vi "Sequencers.vi"() -> ()   [LabVIEW 2019]
panel:
  in  "Elevator Limit Switch":bool
  in  "Adam Smashing the button":bool
  out "Piston 3":bool
  out "Timer Value":i32
  out "Sequencer Step":i32
  out "Piston 2":bool
  out "Piston 1":bool
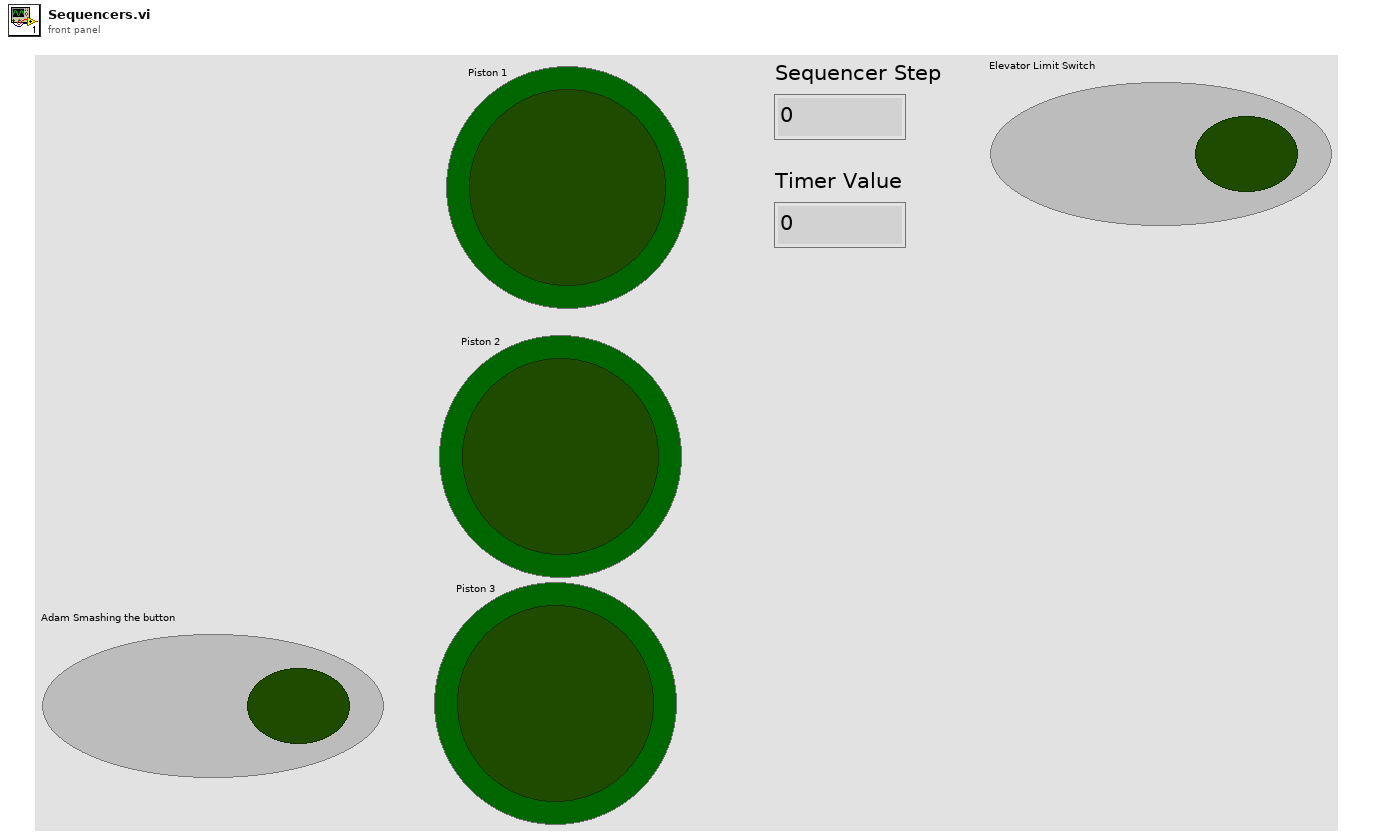
[diagram p1: front panel]
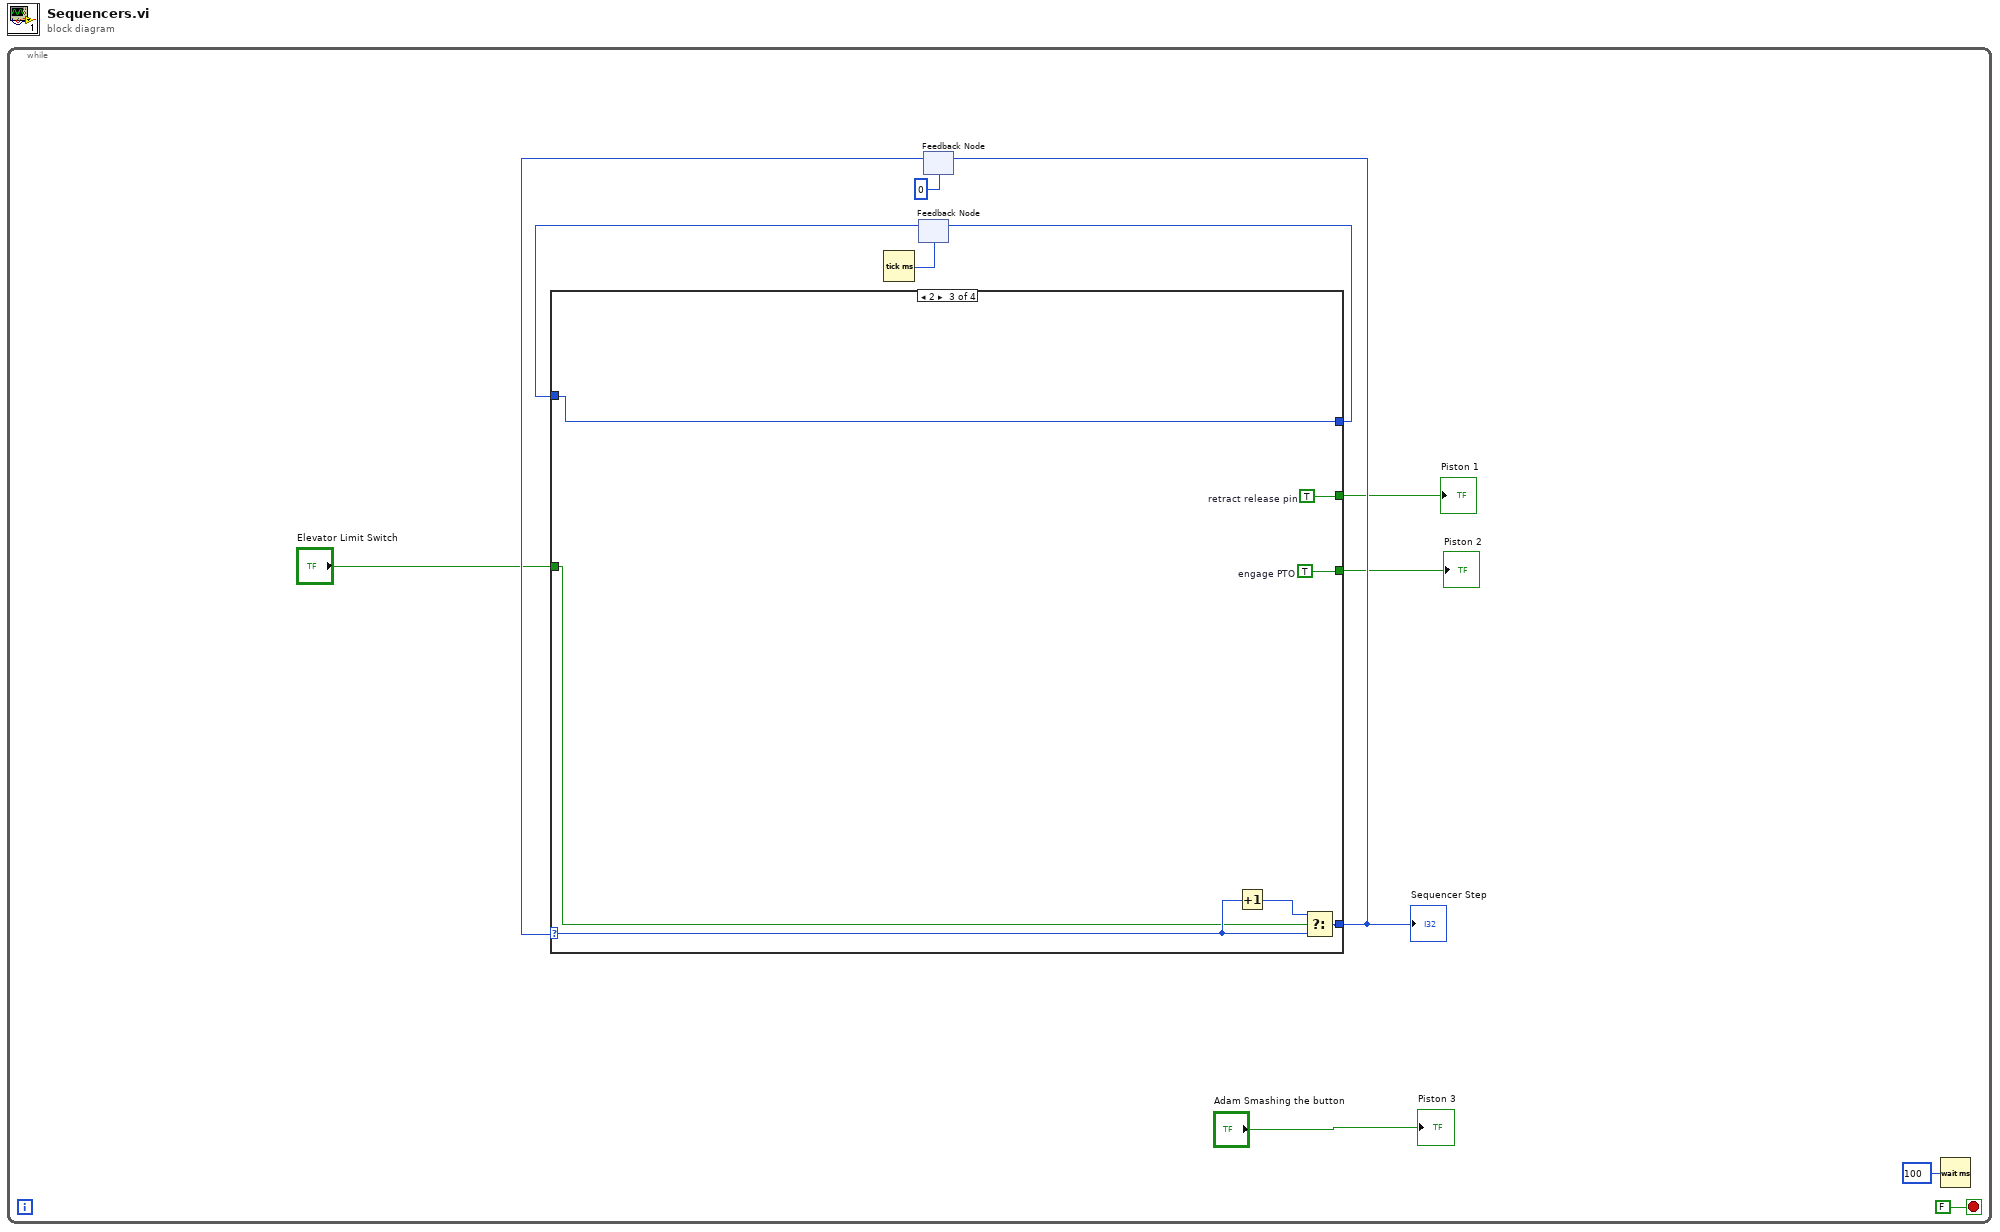
[diagram p0: block diagram]
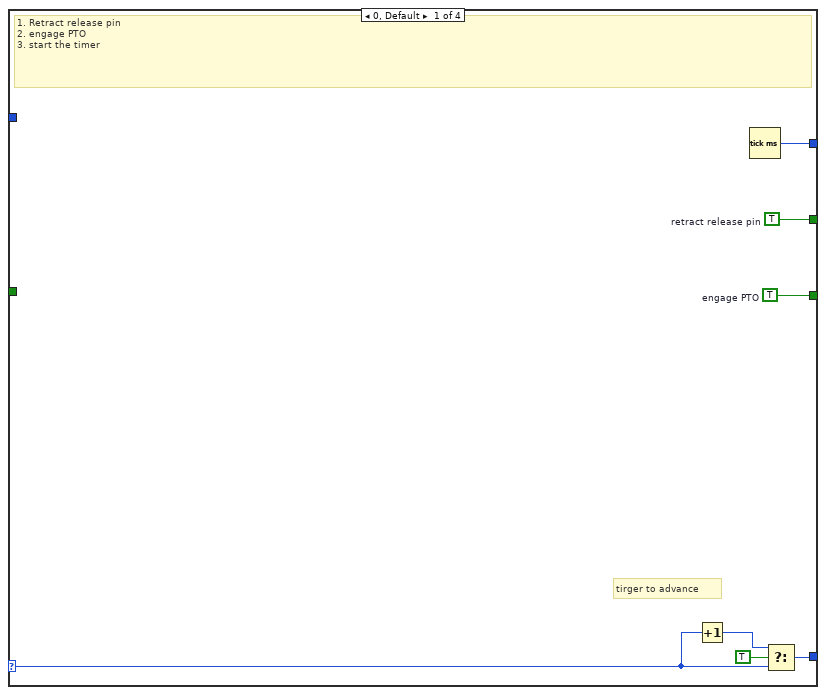
[diagram p2: hidden frame]
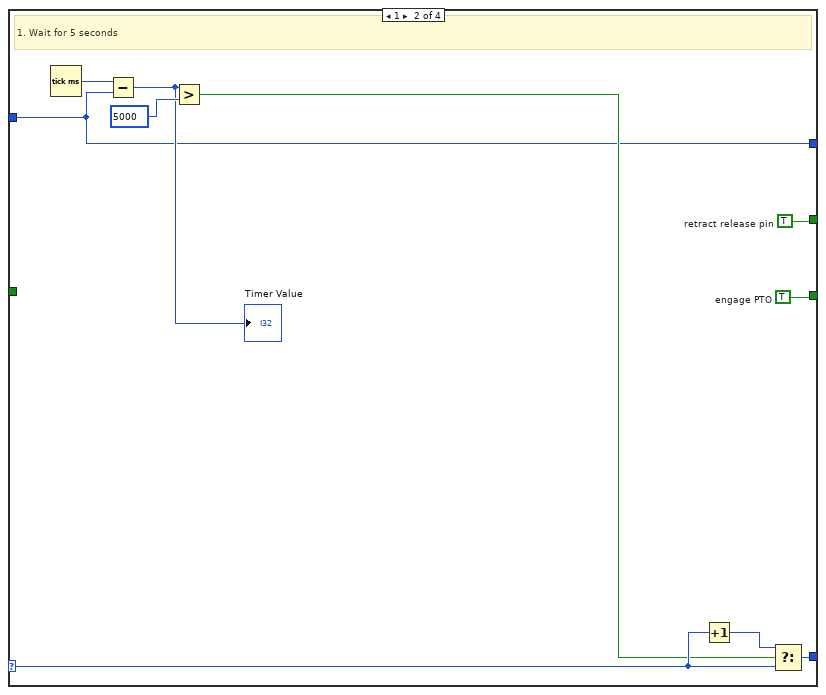
[diagram p3: hidden frame]
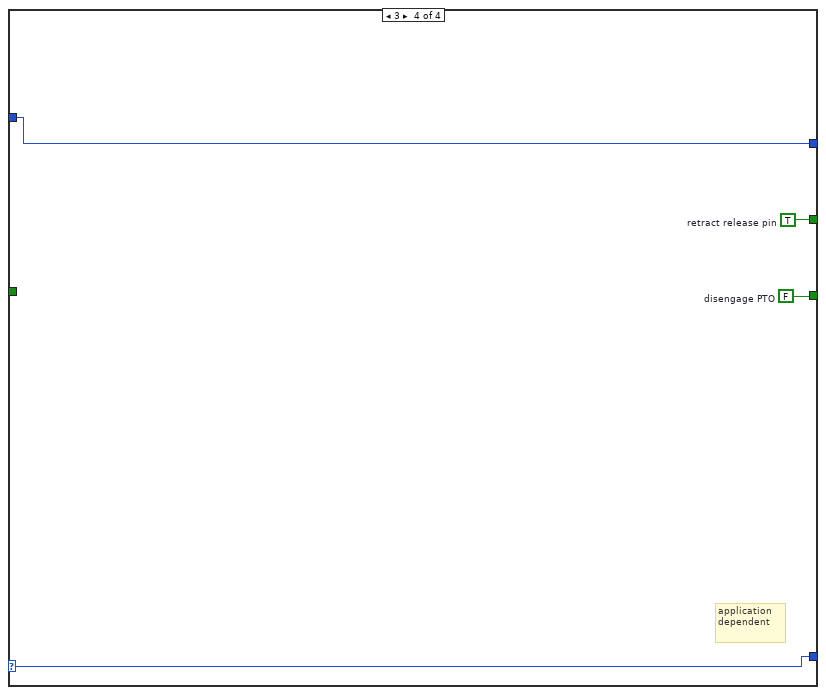
[diagram p4: hidden frame]
diagram:
  n1 = while {
    stop <- FALSE stop-if-true
    n2 = Tick Count (ms)() -> (millisecond timer value=w3:u32)
    n3 = feedback #1(w3) -> (w5:u32)
    n4 = feedback #2(0) -> (w11:i32)
    n5 = case shown="2" w11 {
      selector: w11 -> [w18 w28 w35 w40]
      tunnel: [w19 w27 w34 w40] -> w10
      tunnel: [w16 w26 w33 w39] -> w7
      tunnel: [w15 w25 w32 w38] -> w6
      tunnel: [w13 w20 w31 w37] -> w4
      tunnel: w5 -> [_ w20 w31 w37]
      tunnel: "Elevator Limit Switch" -> [_ _ w30 _]
      frame 0, Default {
        w15 = TRUE  # engage PTO
        w16 = TRUE  # retract release pin
        # "tirger to advance"
        # "1. Retract release pin\n2. engage PTO\n3. start the timer"
        n6 = Increment(x=w18) -> (x+1=w17:i32)
        n7 = Tick Count (ms)() -> (millisecond timer value=w13:u32)
        n8 = Select(t=w17, s=TRUE, f=w18) -> (s? t:f=w19:i32)
      }
      frame 1 {
        w25 = TRUE  # engage PTO
        w26 = TRUE  # retract release pin
        # "1. Wait for 5 seconds"
        n9 = Tick Count (ms)() -> (millisecond timer value=w24:u32)
        n10 = Subtract(x=w24, y=w20) -> (x-y=w21:u32)
        "Timer Value" <- w21
        n11 = Greater?(x=w21, y=u32 5000) -> (0:w22:bool)
        n12 = Increment(x=w28) -> (x+1=w29:i32)
        n13 = Select(t=w29, s=w22, f=w28) -> (s? t:f=w27:i32)
      }
      frame 2 {
        w32 = TRUE  # engage PTO
        w33 = TRUE  # retract release pin
        n14 = Increment(x=w35) -> (x+1=w36:i32)
        n15 = Select(t=w36, s=w30, f=w35) -> (s? t:f=w34:i32)
      }
      frame 3 {
        w38 = FALSE  # disengage PTO
        w39 = TRUE  # retract release pin
        # "application\ndependent"
      }
    }
    "Piston 1" <- w7
    "Piston 2" <- w6
    "Sequencer Step" <- w10
    n16 = feedback-in #1(w4) -> ()
    n17 = feedback-in #2(w10) -> ()
    n18 = Wait (ms)(milliseconds to wait=u32 100) -> ()  [unwired: 1 out]
    "Piston 3" <- "Adam Smashing the button"
  }
